vi "wykladniczy.vi"(11 "lambda":dbl=1.0) -> (3 "X~wykładniczy":dbl)   [LabVIEW 2013, in "LukiBrary.lvlib"]
doc: "Zwraca zmienną losową o rozkładzie wykładniczym."
uses:
  LukiBrary.lvlib
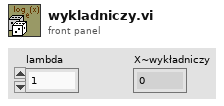
[diagram p1: front panel]
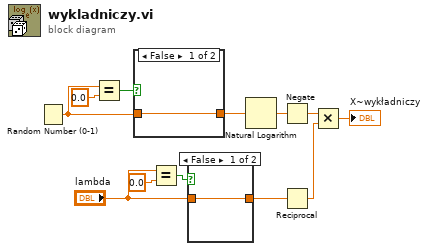
[diagram p0: block diagram]
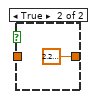
[diagram p2: hidden frame]
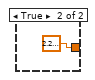
[diagram p3: hidden frame]
diagram:
  n1 = Random Number (0-1)() -> (number: 0 to 1=w10:dbl)
  n2 = Equal?(x=w10, y=0.0) -> (x = y?=w12:bool)
  n3 = case shown="False" w12 {
    tunnel: w10 -> [w13 _]
    tunnel: [w13 2.220446049250313e-16] -> w9
    frame False {
    }
    frame True {
    }
  }
  n4 = Equal?(x="lambda", y=0.0) -> (x = y?=w3:bool)
  n5 = case shown="False" w3 {
    tunnel: "lambda" -> [w15 _]
    tunnel: [w15 2.220446049250313e-16] -> w1
    frame False {
    }
    frame True {
    }
  }
  n6 = Natural Logarithm(1:w9) -> (0:w8:dbl)
  n7 = Negate(x=w8) -> (-x=w7:dbl)
  n8 = Reciprocal(x=w1) -> (1/x=w6:dbl)
  n9 = Multiply(x=w7, y=w6) -> (x*y=→"X~wykładniczy":dbl)
